vi "intialize.vi"(2 "Tolerance (m)":dbl, 3 "Error In":errorcluster) -> (5 "PassBouy.lvclass":refnum<class "PassBouy.lvclass">, 6 "Error Out":errorcluster)   [LabVIEW 2012, in "PassBouy.lvclass"]
doc: "Creates a \"PassBouys\" mission. Given two bouy locations (Port and Starboard), the mission will calculate the waypoints nessisary to guide the boat through the two bouys"
uses:
  PassBouy.lvclass
  Data/TypeDefs/UTM Location.ctl
  Data/TypeDefs/MissionTypeControl.ctl
  PassBouy.lvclass/PassBouy.ctl
panel:
  in  "Starboard":T1 {"North" format="%#_10f"; "East" format="%#_8f"}
  in  "Port":T1 {"North" format="%#_10f"; "East" format="%#_8f"}
  in  "PassBouy.lvclass 2":refnum<class "PassBouy.lvclass">
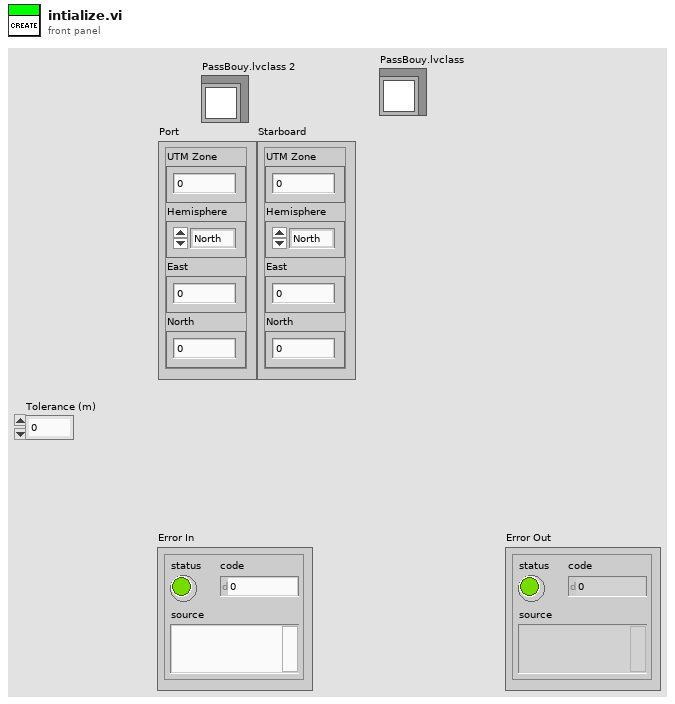
[diagram p1: front panel]
types:
  T1 = typedef "UTM Location.ctl" = cluster{"UTM Zone":dbl, "Hemisphere":enum16{"North", "South"}, "East":dbl, "North":dbl}
  T2 = typedef "MissionTypeControl.ctl" = enum16{"Idle at Point", "Drive to Waypoint", "Round Buoy to Port", "Round Buoy to Starboard", "Pass Between Buoys", "Station Keeping"}
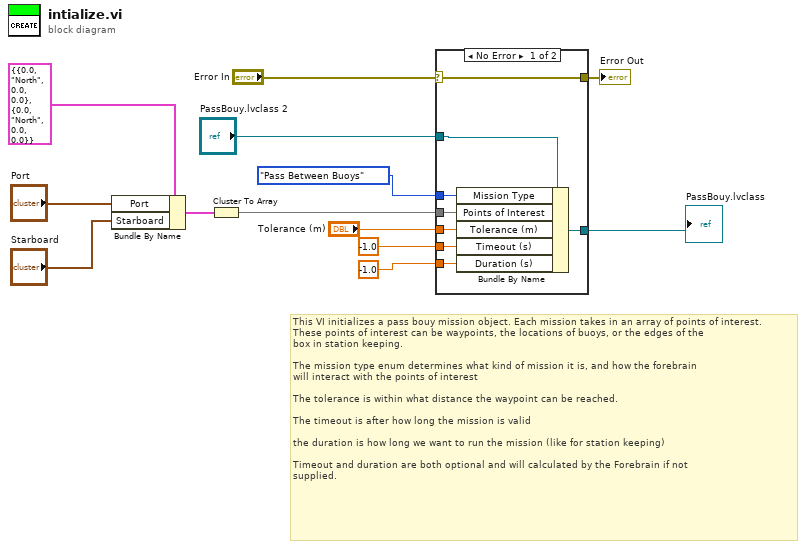
[diagram p0: block diagram]
diagram:
  # "This VI initializes a pass bouy mission object. Each mission takes in an array of points of interest.\nThese points of interest can be waypoints, the locations of buoys, or the edges of the \nbox in station keeping. \n\nThe mission type enum determines what kind of mission it is, and how the forebrain \nwill interact with the points of interest\n\nThe tolerance is within what distance the waypoint can be reached. \n\nThe timeout is after how long the mission is valid\n\nthe duration is how long we want to run the mission (like for station keeping)\n\nTimeout and duration are both optional and will calculated by the Forebrain if not \nsupplied."
  n1 = Bundle By Name(cluster=cluster{"Port":T1, "Starboard":T1} {"Port"={"UTM Zone"=0.0, "Hemisphere"=enum."North", "East"=0.0, "North"=0.0}, "Starboard"={"UTM Zone"=0.0, "Hemisphere"=enum."North", "East"=0.0, "North"=0.0}} ("input cluster"), "Port"="Port", "Starboard"="Starboard") -> (w2:cluster{"Port":T1, "Starboard":T1})
  n2 = Cluster To Array(cluster=w2) -> (array=w1:T1[])
  n3 = case shown="No Error" "Error In" {
    selector: "Error In" -> [w21 w22]
    tunnel: [w21 w22] -> w12
    tunnel: MissionTypeControl."Pass Between Buoys" ("Mission Type") -> [w20 _]
    tunnel: w1 -> [w19 _]
    tunnel: "Tolerance (m)" -> [w18 _]
    tunnel: -1.0 ("Timeout (s)") -> [w17 _]
    tunnel: -1.0 ("Duration (s)") -> [w16 _]
    tunnel: "PassBouy.lvclass 2" -> [w15 w23]
    tunnel: [w14 w23] -> w7
    frame No Error {
      n4 = Bundle By Name(cluster=w15, "Mission Type"=w20, "Points of Interest"=w19, "Tolerance (m)"=w18, "Timeout (s)"=w17, "Duration (s)"=w16) -> (w14:refnum<class "PassBouy.lvclass">)
    }
    frame Error {
    }
  }
  "Error Out" <- w12
  "PassBouy.lvclass" <- w7
